vi "Path to Next X-Y V2015.vi"(5 "Path":i32[][](array[numeric])) -> (0 "Path Out":i32[][](array[numeric]), 1 "X":i32, 2 "Y":i32)   [LabVIEW 2014]
doc: "Deletes the first column of the incoming array and\noutputs first x and y of new incoming array"
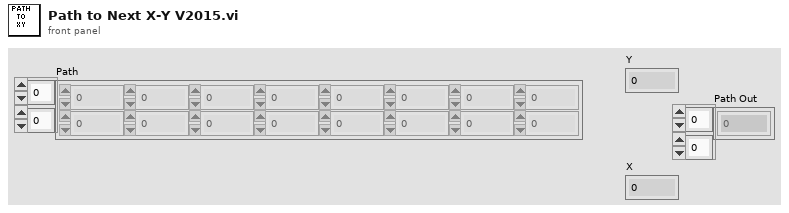
[diagram p1: front panel]
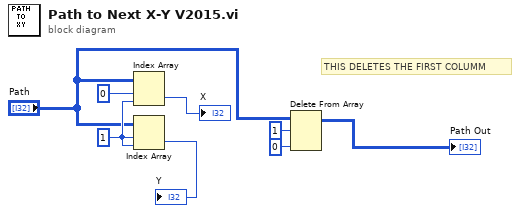
[diagram p0: block diagram]
diagram:
  w5 = 1 ("disabled index (col)")
  # "THIS DELETES THE FIRST COLUMM"
  n1 = Index Array(array="Path", index (row)=0, index (col)=w5) -> (element=→"X":i32)
  n2 = Index Array(array="Path", index (row)=w5, index (col)=w5) -> (element=→"Y":i32)
  n3 = Delete From Array(array="Path", length=1, index (col)=0 ("disabled index (col)")) -> (array with subset deleted=→"Path Out":i32[][])  [unwired: 1 in, 1 out]
